vi "Agilent 34401 Acquire and Graph - SW Triggered.vi"() -> ()   [LabVIEW 2018]
doc: "This example shows how to configure a software triggered measurement using the low-level Data VIs to retrieve data from the DMM.\n\n<B>Note:</B>\n\n(1) It is recommended that all triggered measurements be made using an appropriate fixed manual range. That is, disable autorange and manually select a range in <B>Configure Measurement VI</B>.\n\n(2) To increase the speed of DC measurements, set Autozero to \"once,\" or \"off\" in <B>Configure Autozero VI</B>. \n\n(3) For faster AC measurements, call the Configure AC Filter VI to set the AC filter to 200 Hz, and set the manual trigger delay to 0 seconds in <B>Configure Trigger VI</B>."
uses:
  <vilib>/Utility/error.llb/DialogType.ctl
  <instrlib>/Agilent 34401/Agilent 34401.lvlib
panel:
  in  "Function (0: DC Voltage)":u16(ring) items=["DC Voltage", "AC Voltage", "2 - Wire Resistance", "4 - Wire Resistance", "DC Current", "AC Current", "Frequency", "Period", "Continuity", "Diode Checking", "VDC:VDC Ratio", "Temperature", "Capacitance"]
  in  "Stop":bool
  in  "Manual Range (1.00)":dbl=1.0 format="%_3f"
  in  "Enable Auto Range (F: Disable)":bool
  out "Trigger Iteration":i32
  out "Measurements":dbl[](graph)
  in  "Samples per Trigger (10)":i32=10 format="%#.6g"
  in  "Trigger Count (5)":i32=5 format="%#.6g"
  in  "VISA resource name":refnum<visa-resource-name>
  # "(c) 2005-2015 National Instruments.  ALL RIGHTS RESERVED."
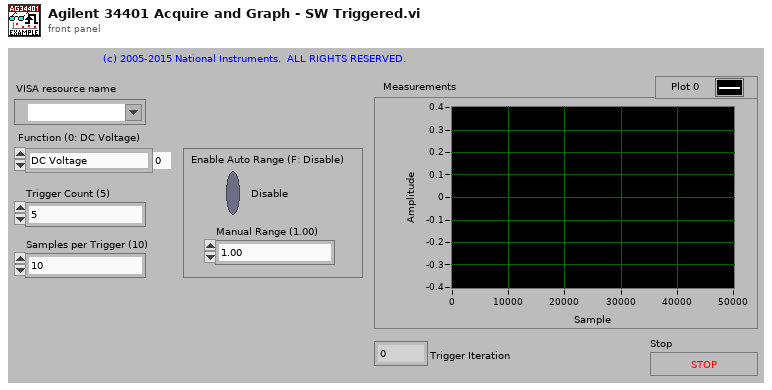
[diagram p1: front panel]
types:
  T1 = typedef "DialogType.ctl" = u16
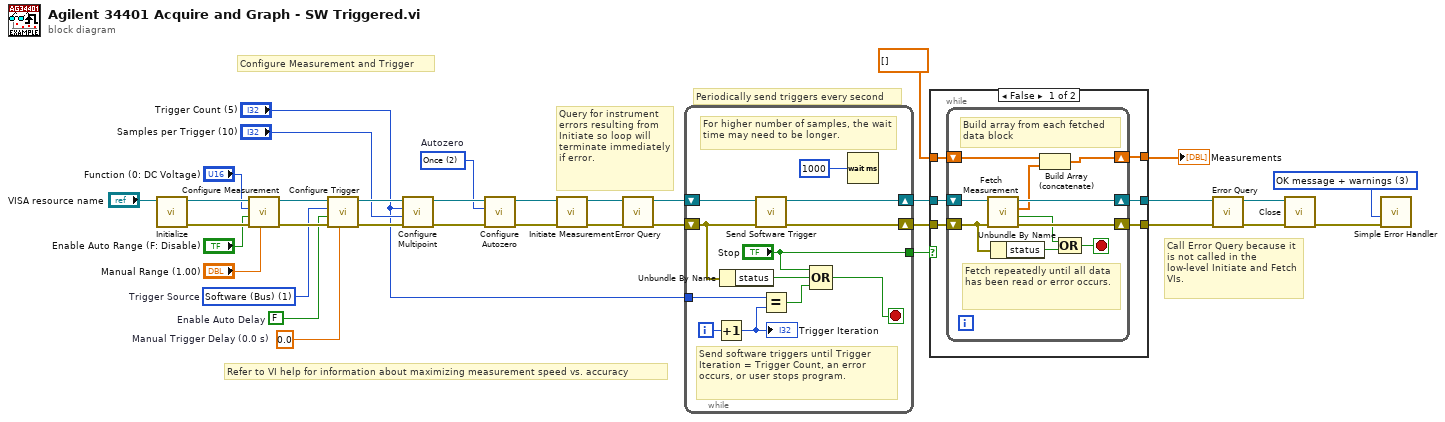
[diagram p0: block diagram]
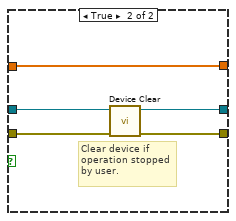
[diagram p2: hidden frame]
diagram:
  w14 = T1 3 items=["no dialog", "OK message", "continue or stop message", "OK message + warnings", "continue/stop + warnings"] ("type of dialog (OK msg:1)")
  w22 = 0.0  # Manual Trigger Delay (0.0 s)
  w23 = u16 2 items=["On", "Off", "Once"]  # Autozero
  w26 = u16 1 items=["Immediate", "Software (Bus)", "External"]  # Trigger Source
  w27 = FALSE  # Enable Auto Delay
  # "Call Error Query because it is not called in the low-level Initiate and Fetch VIs."
  # "Query for instrument errors resulting from Initiate so loop will terminate immediately if error."
  # "Periodically send triggers every second"
  # "Refer to VI help for information about maximizing measurement speed vs. accuracy"
  # "Configure Measurement and Trigger"
  n1 = call <instrlib>:"Initialize.vi"("VISA resource name"="VISA resource name") -> ("error out"=w33:errorcluster, "VISA resource name out"=w34:refnum<visa-resource-name>)  [unwired: 9 in]
  n2 = call <instrlib>:"Configure Measurement.vi"("Manual Range (1.00)"="Manual Range (1.00)", "error in (no error)"=w33, "Enable Auto Range (T: Enable)"="Enable Auto Range (F: Disable)", "Function (0: DC Voltage)"="Function (0: DC Voltage)", "VISA resource name"=w34) -> ("error out"=w31:errorcluster, "VISA resource name out"=w32:refnum<visa-resource-name>)  [unwired: 5 in]
  n3 = call <instrlib>:"Configure Trigger.vi"("Manual Trigger Delay (0.0 s)"=w22, "error in (no error)"=w31, "Enable Auto Delay (T: Enable)"=w27, "Trigger Source (0: Immediate)"=w26, "VISA resource name"=w32) -> ("error out"=w29:errorcluster, "VISA resource name out"=w30:refnum<visa-resource-name>)  [unwired: 5 in]
  n4 = call <instrlib>:"Configure Multipoint.vi"("error in (no error)"=w29, "Sample Count (1)"="Samples per Trigger (10)", "Trigger Count (1)"="Trigger Count (5)", "VISA resource name"=w30) -> ("error out"=w25:errorcluster, "VISA resource name out"=w24:refnum<visa-resource-name>)  [unwired: 6 in]
  n5 = call <instrlib>:"Configure Autozero.vi"("error in (no error)"=w25, "Autozero  (0: On)"=w23, "VISA resource name"=w24) -> ("error out"=w21:errorcluster, "VISA resource name out"=w20:refnum<visa-resource-name>)  [unwired: 7 in]
  n6 = call <instrlib>:"Initiate Measurement.vi"("error in (no error)"=w21, "VISA resource name"=w20) -> ("error out"=w12:errorcluster, "VISA resource name out"=w11:refnum<visa-resource-name>)  [unwired: 8 in]
  n7 = call <instrlib>:"Error Query.vi"("error in (no error)"=w12, "VISA resource name"=w11) -> ("error out"=w9:errorcluster, "VISA resource name out"=w10:refnum<visa-resource-name>)  [unwired: 6 in, 2 out]
  n8 = while {
    shift-right: [w46] -> w18
    shift-left: w9 -> [w42]
    shift-right: [w45] -> w19
    shift-left: w10 -> [w47]
    tunnel: "Trigger Count (5)" -> [w40]
    tunnel: ["Stop"] -> w7
    i -> [w43]
    stop <- w37 stop-if-true
    # "Send software triggers until Trigger Iteration = Trigger Count, an error occurs, or user stops program."
    # "For higher number of samples, the wait time may need to be longer."
    n9 = Increment(x=w43) -> (x+1=w41:i32)
    "Trigger Iteration" <- w41
    n10 = Unbundle By Name(w42) -> ("status"=w39:bool)
    n11 = call <instrlib>:"Send Software Trigger.vi"("error in (no error)"=w42, "VISA resource name"=w47) -> ("error out"=w46:errorcluster, "VISA resource name out"=w45:refnum<visa-resource-name>)  [unwired: 8 in]
    n12 = Equal?(x=w40, y=w41) -> (x = y?=w38:bool)
    n13 = Compound Arithmetic op=OR("Stop", w39, w38) -> (w37:bool)
    n14 = Wait (ms)(milliseconds to wait=u32 1000 ("millisecond multiple")) -> ()  [unwired: 1 out]
  }
  n15 = case shown="False" w7 {
    tunnel: w19 -> [w53 w67]
    tunnel: w18 -> [w52 w68]
    tunnel: [w49 w64] -> w17
    tunnel: [w51 w66] -> w3
    tunnel: [w50 w65] -> w2
    tunnel: dbl[] [] -> [w48 w64]
    frame False {
      n16 = while {
        shift-right: [w58] -> w49
        shift-left: w48 -> [w59]
        shift-right: [w61] -> w50
        shift-left: w52 -> [w57]
        shift-right: [w62] -> w51
        shift-left: w53 -> [w63]
        stop <- w54 stop-if-true
        # "Build array from each fetched data block"
        # "Fetch repeatedly until all data has been read or error occurs."
        n17 = call <instrlib>:"Fetch Measurement.vi"("error in (no error)"=w57, "VISA resource name"=w63) -> ("error out"=w61:errorcluster, "End of Data?"=w56:bool, "Measurements"=w60:dbl[], "VISA resource name out"=w62:refnum<visa-resource-name>)  [unwired: 6 in]
        n18 = Unbundle By Name(w57) -> ("status"=w55:bool)
        n19 = Build Array (concatenate)(w59, w60) -> (w58:dbl[])
        n20 = Compound Arithmetic op=OR(w56, w55) -> (w54:bool)
      }
    }
    frame True {
      # "Clear device if operation stopped by user."
      n21 = call <instrlib>:"Device Clear.vi"("error in (no error)"=w68, "VISA Resource Name"=w67) -> ("error out"=w65:errorcluster, "VISA Resource Out"=w66:refnum<visa-resource-name>)  [unwired: 8 in]
    }
  }
  "Measurements" <- w17
  n22 = call <instrlib>:"Error Query.vi"("error in (no error)"=w2, "VISA resource name"=w3) -> ("error out"=w5:errorcluster, "VISA resource name out"=w4:refnum<visa-resource-name>)  [unwired: 6 in, 2 out]
  n23 = call <instrlib>:"Close.vi"("error in (no error)"=w5, "VISA resource name"=w4) -> ("error out"=w28:errorcluster)  [unwired: 9 in]
  n24 = call <vilib>:"Simple Error Handler.vi"("type of dialog (OK msg:1)"=w14, "error in (no error)"=w28) -> ()  [unwired: 3 in, 5 out]
